vi "filter gradient.vi"(6 "Threshold":dbl=2.0, 7 "Weights type":u16(ring)=1 items=["None", "G", "G^2"], 8 "Threshold type":u16(ring) items=["Top fraction", "Top value"], 9 "Gy":dbl[][](array[numeric]), 10 "Gx":dbl[][](array[numeric]), 11 "G":dbl[][](array[numeric])) -> (0 "Weights":dbl[](array[numeric]), 1 "gradients":dbl[][](array[numeric]), 2 "centers":i32[][](array[numeric]), 3 "Filtered G":dbl[][](graph), 4 "Threshold out":dbl, 5 "Mask":i16[][](array[numeric]))   [LabVIEW 2015]
doc: "Filters input local gradient images by magnitude of the gradient. Also returns arrays for least square fitting.\n\nINPUT\nG,Gx,Gy - magnitude, horizontal and vertical local gradients correspondingly.\nThreshold type, - type of threshold to apply:\n\"Top fraction\" - sets threshold as max_intensity/Threshold, e.g., for a Threshold=2 the threshold will be set to half the maximum pixel value \n\"Top value\" - sets the threshold to Threshold\nThreshold - threshold value\n\nOUTPUT\nFiltered G - filtered magnitude of the gradient\nMask\ncenters - pixel centers (2 column array)\ngradients - gradients (2 column array)\nWeights - gradient line weights (1D array)\n\nAuthor: Anatolii Kashchuk"
panel:
  # "Author: Anatolii Kashchuk"
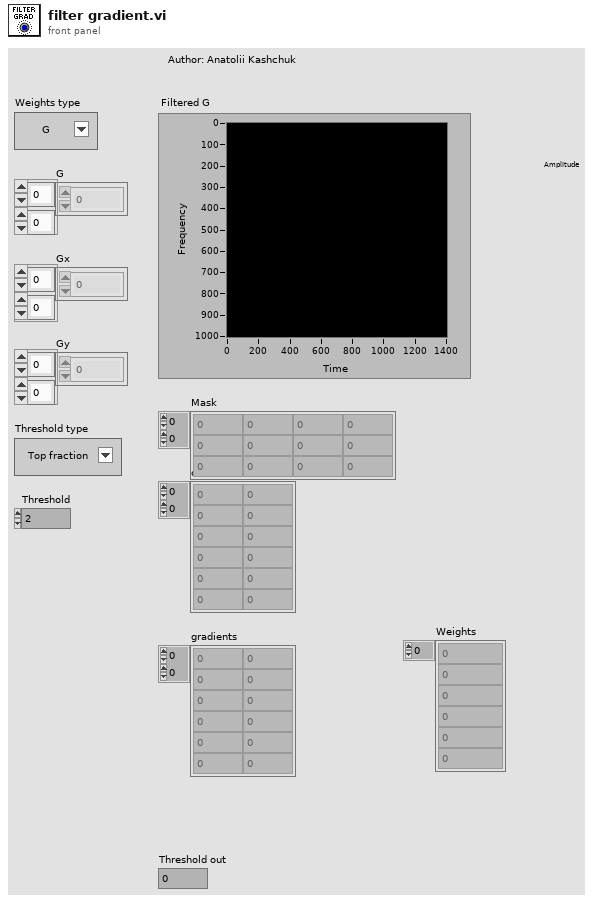
[diagram p1: front panel]
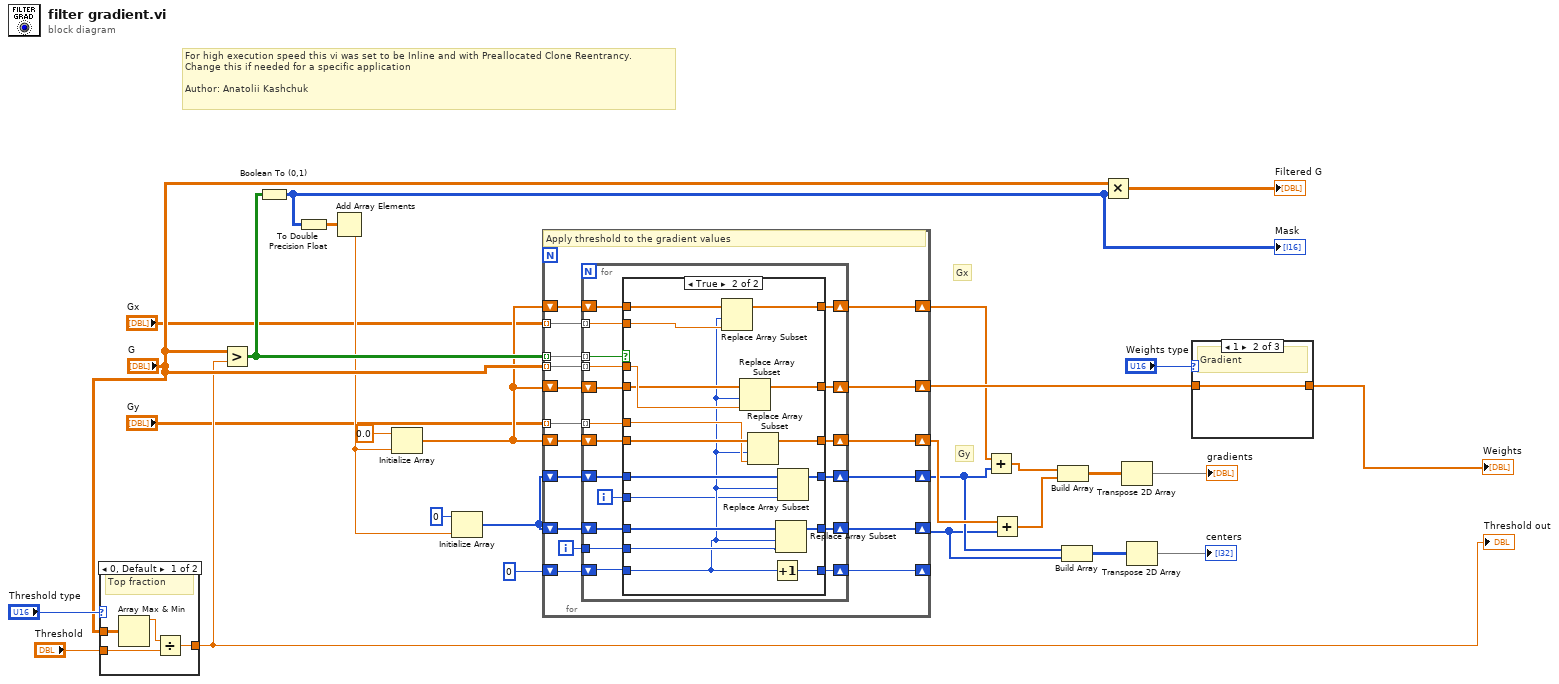
[diagram p0: block diagram]
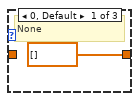
[diagram p3: hidden frame]
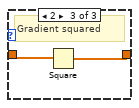
[diagram p4: hidden frame]
diagram:
  # "For high execution speed this vi was set to be Inline and with Preallocated Clone Reentrancy. \nChange this if needed for a specific application\n\nAuthor: Anatolii Kashchuk"
  # "Gy"
  # "Gx"
  n1 = case shown="0, Default" "Threshold type" {
    tunnel: "Threshold" -> [w33 w34]
    tunnel: [w31 w34] -> w23
    tunnel: "G" -> [w30 _]
    frame 0, Default {
      # "Top fraction"
      n2 = Array Max & Min(array=w30) -> (max value=w32:dbl)  [unwired: 3 out]
      n3 = Divide(x=w32, y=w33) -> (x/y=w31:dbl)
    }
    frame 1 {
      # "Top value"
    }
  }
  "Threshold out" <- w23
  n4 = Greater?(x="G", y=w23) -> (0:w22:bool[][])
  n5 = Boolean To (0,1)(Boolean=w22) -> (0, 1=w1:i16[][])
  "Mask" <- w1
  n6 = To Double Precision Float(number=w1) -> (double precision float=w2:dbl[][])
  n7 = Add Array Elements(numeric array=w2) -> (sum=w19:dbl)
  n8 = Initialize Array(0.0, w19) -> (w17:dbl[])
  n9 = Initialize Array(0, w19) -> (w13:i32[])
  n10 = for {
    tunnel: "G" -> [w51] mode=indexing
    tunnel: "Gx" -> [w50] mode=indexing
    tunnel: w22 -> [w49] mode=indexing
    shift-right: [w47] -> w10
    shift-left: w17 -> [w48]
    shift-right: [w45] -> w12
    shift-left: w17 -> [w46]
    shift-right: [w42] -> w7
    shift-left: w13 -> [w43]
    shift-right: [w40] -> _
    shift-left: 0 -> [w41]
    tunnel: "Gy" -> [w39] mode=indexing
    shift-right: [w37] -> w14
    shift-left: w17 -> [w38]
    shift-right: [w35] -> w8
    shift-left: w13 -> [w36]
    i -> [w44]
    # "Apply threshold to the gradient values"
    n11 = for {
      tunnel: w51 -> [w56] mode=indexing
      tunnel: w50 -> [w57] mode=indexing
      tunnel: w49 -> [w68] mode=indexing
      shift-right: [w66] -> w47
      shift-left: w48 -> [w67]
      shift-right: [w64] -> w45
      shift-left: w46 -> [w65]
      tunnel: w44 -> [w63]
      shift-right: [w61] -> w42
      shift-left: w43 -> [w62]
      shift-right: [w59] -> w40
      shift-left: w41 -> [w60]
      tunnel: w39 -> [w58] mode=indexing
      shift-right: [w54] -> w37
      shift-left: w38 -> [w55]
      shift-right: [w52] -> w35
      shift-left: w36 -> [w53]
      i -> [w69]
      n12 = case shown="True" w68 {
        tunnel: w69 -> [_ w76]
        tunnel: w67 -> [w75 w92]
        tunnel: [w75 w91] -> w66
        tunnel: w65 -> [w74 w90]
        tunnel: [w74 w84] -> w64
        tunnel: w58 -> [_ w86]
        tunnel: w63 -> [_ w80]
        tunnel: w62 -> [w73 w89]
        tunnel: [w73 w88] -> w61
        tunnel: w60 -> [w72 w77]
        tunnel: [w72 w87] -> w59
        tunnel: w57 -> [_ w85]
        tunnel: w56 -> [_ w83]
        tunnel: w55 -> [w71 w82]
        tunnel: [w71 w81] -> w54
        tunnel: w53 -> [w70 w79]
        tunnel: [w70 w78] -> w52
        frame False {
        }
        frame True {
          n13 = Replace Array Subset(array=w90, new element=w85, index=w77) -> (w84:dbl[])
          n14 = Replace Array Subset(array=w82, new element=w83, index=w77) -> (w81:dbl[])
          n15 = Replace Array Subset(array=w92, new element=w86, index=w77) -> (w91:dbl[])
          n16 = Increment(x=w77) -> (x+1=w87:i32)
          n17 = Replace Array Subset(array=w89, new element=w80, index=w77) -> (w88:i32[])
          n18 = Replace Array Subset(array=w79, new element=w76, index=w77) -> (w78:i32[])
        }
      }
    }
  }
  n19 = Add(x=w12, y=w8) -> (x+y=w11:dbl[])
  n20 = Add(x=w10, y=w7) -> (x+y=w9:dbl[])
  n21 = Build Array(w11, w9) -> (w5:dbl[][])
  n22 = Build Array(w8, w7) -> (w6:i32[][])
  n23 = Multiply(x="G", y=w1) -> (x*y=→"Filtered G":dbl[][])
  n24 = Transpose 2D Array(2D array=w5) -> (transposed array=→"gradients":dbl[][])
  n25 = Transpose 2D Array(2D array=w6) -> (transposed array=→"centers":i32[][])
  n26 = case shown="1" "Weights type" {
    tunnel: w14 -> [_ w94 w96]
    tunnel: [dbl[] [] w94 w95] -> w25
    frame 0, Default {
      # "None"
    }
    frame 1 {
      # "Gradient"
    }
    frame 2 {
      # "Gradient squared"
      n27 = Square(x=w96) -> (x^2=w95:dbl[])
    }
  }
  "Weights" <- w25
